vi "create scan vectr.vi"(1 "Table Control":string[][](table)) -> (0 "Array":dbl[](array[numeric]))   [LabVIEW 2017]
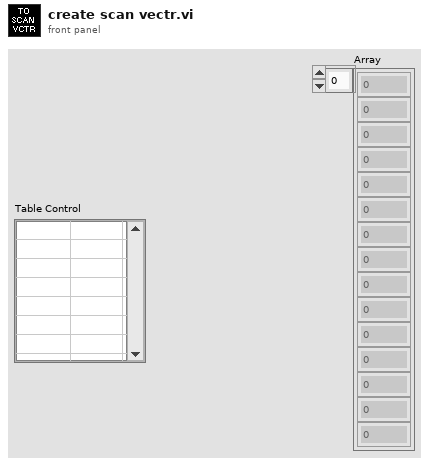
[diagram p1: front panel]
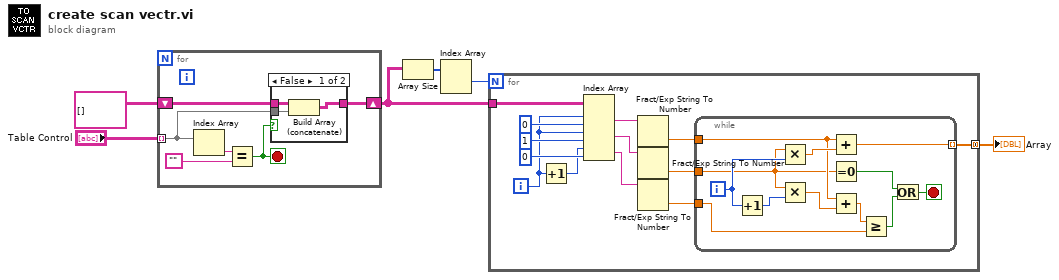
[diagram p0: block diagram]
diagram:
  n1 = for {
    tunnel: "Table Control" -> [w8] mode=indexing
    shift-right: [w7] -> w3
    shift-left: string[][] [] ("t") -> [w10]
    stop <- w9 stop-if-true
    n2 = Index Array(array=w8) -> (element=w11:string)  [unwired: 1 in]
    n3 = Equal?(x=w11, y="") -> (x = y?=w9:bool)
    n4 = case shown="False" w9 {
      tunnel: w10 -> [w15 w16]
      tunnel: w8 -> [w14 _]
      tunnel: [w13 w16] -> w7
      frame False {
        n5 = Build Array (concatenate)(w15, w14) -> (w13:string[][])
      }
      frame True {
      }
    }
  }
  n6 = Array Size(array=w3) -> (size(s)=w6:i32[])
  n7 = Index Array(array=w6) -> (element #1=w2:i32)  [unwired: 2 in, 1 out]
  n8 = for {
    N: w2 -> [_]
    tunnel: w3 -> [w25]
    tunnel: [w17] -> w1 mode=concatenating
    i -> [w24]
    n9 = Increment(x=w24) -> (x+1=w27:i32)
    n10 = Index Array(array=w25, index (row) #1=w24, index (col) #1=0 ("disabled index (col)"), index (row) #2=w24, index (col) #2=1 ("disabled index (col)"), index (row) #3=w27, index (col) #3=0 ("disabled index (col)")) -> (element #1=w23:string, element #2=w22:string, element #3=w21:string)
    n11 = Fract/Exp String To Number(string=w23) -> (number=w20:dbl)  [unwired: 3 in, 1 out]
    n12 = Fract/Exp String To Number(string=w22) -> (number=w19:dbl)  [unwired: 3 in, 1 out]
    n13 = Fract/Exp String To Number(string=w21) -> (number=w18:dbl)  [unwired: 3 in, 1 out]
    n14 = while {
      tunnel: w20 -> [w36]
      tunnel: w19 -> [w33]
      tunnel: w18 -> [w34]
      tunnel: [w40] -> w17 mode=indexing
      i -> [w38]
      stop <- w30 stop-if-true
      n15 = Increment(x=w38) -> (x+1=w37:i32)
      n16 = Multiply(x=w33, y=w38) -> (x*y=w41:dbl)
      n17 = Multiply(x=w33, y=w37) -> (x*y=w39:dbl)
      n18 = Add(x=w36, y=w41) -> (x+y=w40:dbl)
      n19 = Equal To 0?(x=w33) -> (x = 0?=w32:bool)
      n20 = Add(x=w36, y=w39) -> (x+y=w35:dbl)
      n21 = Greater Or Equal?(x=w35, y=w34) -> (x >= y?=w31:bool)
      n22 = Or(x=w32, y=w31) -> (x .or. y?=w30:bool)
    }
  }
  "Array" <- w1
